vi "Set Data.vi"(0 "2D Double Data in":refnum<class "2D Double Logging Data.lvclass">, 5 "Group Name":string, 7 "Channel Names":string[](array[string]), 9 "Data":dbl[][](array[numeric]), 11 "error in (no error)":errorcluster) -> (4 "2D Double Data out":refnum<class "2D Double Logging Data.lvclass">, 15 "error out":errorcluster)   [LabVIEW 2024, in "Logging Data.lvlib" / "2D Double Logging Data.lvclass"]
uses:
  2D Double Logging Data.lvclass
  C:/Users/uspoaotto/OneDrive - Oregon Tool/Desktop/working copies/dataLogger/Logging Data/Logging Data/Logging Data.lvclass
  2D Double Logging Data.lvclass/2D Double Logging Data.ctl
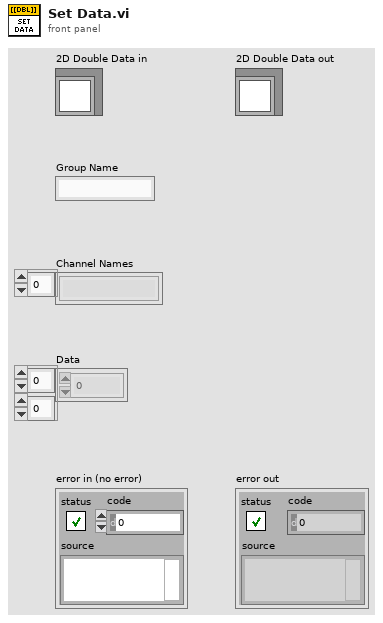
[diagram p1: front panel]
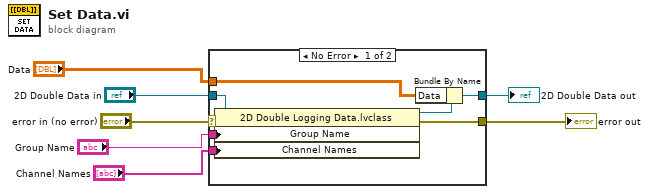
[diagram p0: block diagram]
diagram:
  n1 = case shown="No Error" "error in (no error)" {
    selector: "error in (no error)" -> [w10 w17]
    tunnel: [w8 w17] -> w6
    tunnel: [w9 w16] -> w4
    tunnel: "2D Double Data in" -> [w15 w16]
    tunnel: "Data" -> [w13 _]
    tunnel: "Group Name" -> [w12 _]
    tunnel: "Channel Names" -> [w11 _]
    frame No Error {
      n2 = property class="2D Double Logging Data.lvclass"(reference=w15, error in=w10, "Group Name"=w12, "Channel Names"=w11) -> (reference out=w14:refnum<class "2D Double Logging Data.lvclass">, error out=w8:errorcluster)
      n3 = Bundle By Name(cluster=w14, "Data"=w13) -> (w9:refnum<class "2D Double Logging Data.lvclass">)
    }
    frame Error {
    }
  }
  "error out" <- w6
  "2D Double Data out" <- w4
